vi "ApplicationControlView.vi"(10 "Communicator":refnum<class "Communicator.lvclass">, 11 "UserEvents":refnum<class "UserEvents.lvclass">) -> ()   [LabVIEW 2016, in "M1M3SupportViews.lvlib"]
uses:
  M1M3SupportViews.lvlib
  UserEvents/UserEvents.lvclass
  Communicator/Communicator/Communicator.lvclass
  UserEvents/UserEvents.lvclass/UserEvents.ctl
  DataTypes/Topics/Parts/SummaryStates.ctl
  DataTypes/Topics/CommandStart.ctl
  DataTypes/Topics/Parts/CommandId.ctl
  DataTypes/Topics/CommandEnable.ctl
  DataTypes/Topics/CommandDisable.ctl
  DataTypes/Topics/CommandStandby.ctl
  DataTypes/General/ShutdownEvent.ctl
  DataTypes/Topics/CommandExit.ctl
  DataTypes/Topics/M1M3SupportTopics.lvlib
  DataTypes/General/M1M3SupportGeneral.lvlib
panel:
  in  "Exit":bool
  in  "Shutdown":bool
  in  "Standby":bool
  in  "Disable":bool
  in  "Enable":bool
  in  "Start":bool
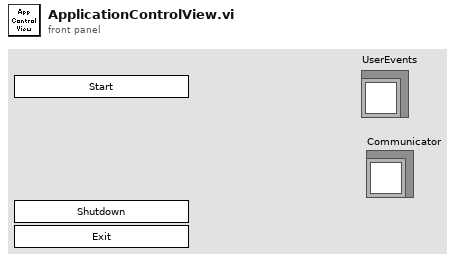
[diagram p1: front panel]
types:
  T1 = typedef "M1M3SupportTopics.lvlib/SummaryStates.ctl" = enum16{"OfflineState", "StandbyState", "DisabledState", "EnabledState", "FaultState"}
  T2 = typedef "M1M3SupportTopics.lvlib/CommandStart.ctl" = cluster{"CommandId":T3, "Start":bool, "SettingToApply":string}
  T3 = typedef "M1M3SupportTopics.lvlib/CommandId.ctl" = i32
  T4 = typedef "M1M3SupportTopics.lvlib/CommandEnable.ctl" = cluster{"CommandId":T3, "Enable":bool}
  T5 = typedef "M1M3SupportTopics.lvlib/CommandDisable.ctl" = cluster{"CommandId":T3, "Disable":bool}
  T6 = typedef "M1M3SupportTopics.lvlib/CommandStandby.ctl" = cluster{"CommandId":T3, "Standby":bool}
  T7 = typedef "M1M3SupportGeneral.lvlib/ShutdownEvent.ctl" = cluster{"Shutdown":bool}
  T8 = typedef "M1M3SupportTopics.lvlib/CommandExit.ctl" = cluster{"CommandId":T3, "Exit":bool}
  T9 = typedef "M1M3SupportTypes.lvlib/SummaryStates.ctl" = enum16{"OfflineState", "StandbyState", "DisabledState", "EnabledState", "FaultState"}
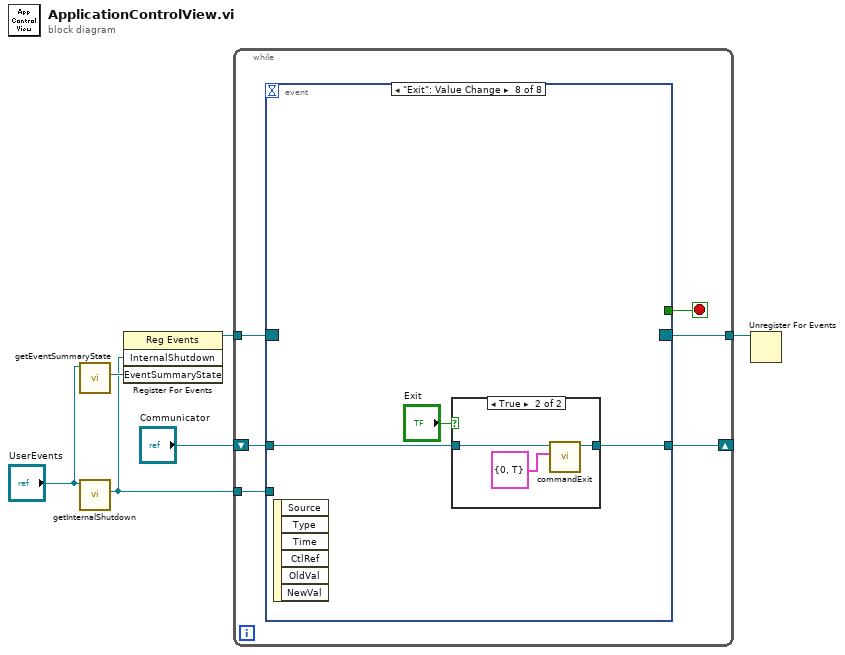
[diagram p0: block diagram]
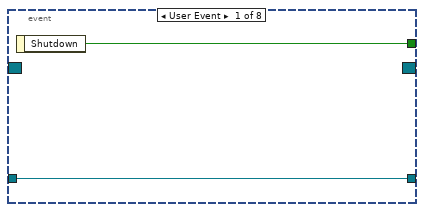
[diagram p2: hidden frame]
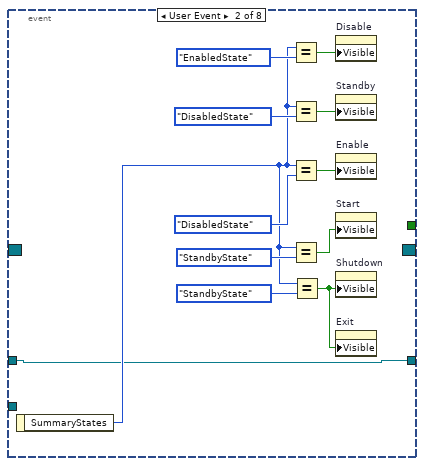
[diagram p3: hidden frame]
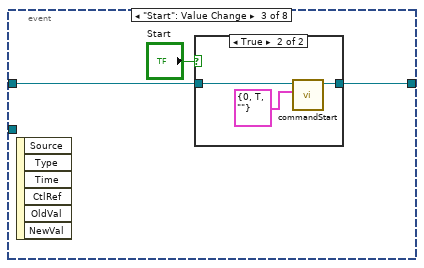
[diagram p4: hidden frame]
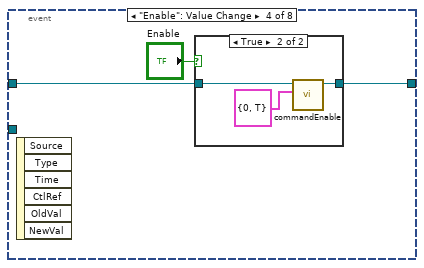
[diagram p6: hidden frame]
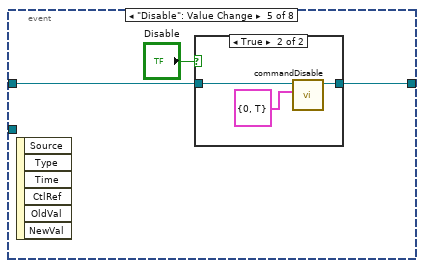
[diagram p8: hidden frame]
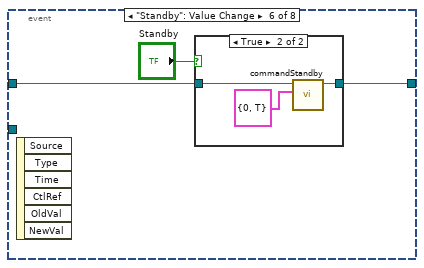
[diagram p10: hidden frame]
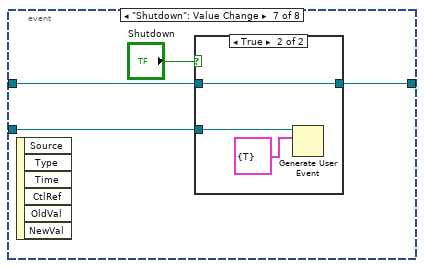
[diagram p12: hidden frame]
diagram:
  n1 = call "getEventSummaryState.vi"("UserEvents in"="UserEvents") -> ("EventSummaryState"=w6:refnum<user-event>)  [unwired: 9 in, 1 out]
  n2 = call "getInternalShutdown.vi"("UserEvents in"="UserEvents") -> ("InternalShutdown"=w1:refnum<user-event>)  [unwired: 9 in, 1 out]
  n3 = register-events(w1, w6) -> (reference out=w5:refnum<event-registration>)  [unwired: 2 in, 1 out]
  n4 = while {
    tunnel: w5 -> [w12]
    tunnel: [w11] -> w4
    shift-right: [w8] -> _
    shift-left: "Communicator" -> [w9]
    tunnel: w1 -> [w7]
    stop <- w10 stop-if-true
    n5 = event shown="[7] \"Exit\": Value Change" {
      selector: w12 -> [_ _ _ _ _ _ _ _]
      dyn-events: [_ _ _ _ _ _ _ _] -> w11
      timeout: _ -> [_ _ _ _ _ _ _ _]
      tunnel: [w14 _ _ _ _ _ _ _] -> w10
      tunnel: w9 -> [w13 w16 w29 w36 w43 w50 w58 w65]
      tunnel: [w13 w16 w28 w35 w42 w49 w57 w64] -> w8
      tunnel: w7 -> [_ _ _ _ _ _ w55 _]
      event User Event {
        n6 = event-data() -> ("Shutdown"=w14:bool)  [unwired: 1 in]
      }
      event User Event {
        n7 = event-data() -> ("SummaryStates"=w17:T9)  [unwired: 1 in]
        n8 = Equal?(x=w17, y=SummaryStates."EnabledState") -> (x = y?=w19:bool)
        n9 = Equal?(x=w17, y=SummaryStates."DisabledState") -> (x = y?=w20:bool)
        n10 = Equal?(x=w17, y=SummaryStates."DisabledState") -> (x = y?=w23:bool)
        n11 = Equal?(x=w17, y=SummaryStates."StandbyState") -> (x = y?=w24:bool)
        n12 = Equal?(x=w17, y=SummaryStates."StandbyState") -> (x = y?=w15:bool)
        n13 = property on="Disable" class="Bool"("Visible"=w19) -> ()  [unwired: 2 in, 2 out]
        n14 = property on="Standby" class="Bool"("Visible"=w20) -> ()  [unwired: 2 in, 2 out]
        n15 = property on="Enable" class="Bool"("Visible"=w23) -> ()  [unwired: 2 in, 2 out]
        n16 = property on="Start" class="Bool"("Visible"=w24) -> ()  [unwired: 2 in, 2 out]
        n17 = property on="Shutdown" class="Bool"("Visible"=w15) -> ()  [unwired: 2 in, 2 out]
        n18 = property on="Exit" class="Bool"("Visible"=w15) -> ()  [unwired: 2 in, 2 out]
      }
      event "Start": Value Change {
        n19 = event-data() -> ()  [unwired: 1 in, 6 out]
        n20 = case shown="True" "Start" {
          tunnel: w29 -> [w30 w32]
          tunnel: [w30 w31] -> w28
          frame False {
          }
          frame True {
            n21 = call-dynamic "commandStart.vi"("CommandStart in"=T2 {"CommandId"=0, "Start"=TRUE, "SettingToApply"=""} ("CommandEnterControl in"), "Communicator in"=w32) -> ("Communicator out"=w31:refnum<class "Communicator.lvclass">)  [unwired: 7 in, 2 out]
          }
        }
      }
      event "Enable": Value Change {
        n22 = event-data() -> ()  [unwired: 1 in, 6 out]
        n23 = case shown="True" "Enable" {
          tunnel: w36 -> [w37 w39]
          tunnel: [w37 w38] -> w35
          frame False {
          }
          frame True {
            n24 = call-dynamic "commandEnable.vi"("CommandEnable in"=T4 {"CommandId"=0, "Enable"=TRUE} ("CommandEnterControl in"), "Communicator in"=w39) -> ("Communicator out"=w38:refnum<class "Communicator.lvclass">)  [unwired: 7 in, 2 out]
          }
        }
      }
      event "Disable": Value Change {
        n25 = event-data() -> ()  [unwired: 1 in, 6 out]
        n26 = case shown="True" "Disable" {
          tunnel: w43 -> [w44 w46]
          tunnel: [w44 w45] -> w42
          frame False {
          }
          frame True {
            n27 = call-dynamic "commandDisable.vi"("CommandDisable in"=T5 {"CommandId"=0, "Disable"=TRUE} ("CommandEnterControl in"), "Communicator in"=w46) -> ("Communicator out"=w45:refnum<class "Communicator.lvclass">)  [unwired: 7 in, 2 out]
          }
        }
      }
      event "Standby": Value Change {
        n28 = event-data() -> ()  [unwired: 1 in, 6 out]
        n29 = case shown="True" "Standby" {
          tunnel: w50 -> [w51 w53]
          tunnel: [w51 w52] -> w49
          frame False {
          }
          frame True {
            n30 = call-dynamic "commandStandby.vi"("CommandStandby in"=T6 {"CommandId"=0, "Standby"=TRUE} ("CommandEnterControl in"), "Communicator in"=w53) -> ("Communicator out"=w52:refnum<class "Communicator.lvclass">)  [unwired: 7 in, 2 out]
          }
        }
      }
      event "Shutdown": Value Change {
        n31 = event-data() -> ()  [unwired: 1 in, 6 out]
        n32 = case shown="True" "Shutdown" {
          tunnel: w58 -> [w59 w60]
          tunnel: [w59 w60] -> w57
          tunnel: w55 -> [_ w62]
          frame False {
          }
          frame True {
            n33 = Generate User Event(user event=w62, event data cluster=T7 {"Shutdown"=TRUE} ("event data")) -> ()  [unwired: 2 in, 2 out]
          }
        }
      }
      event "Exit": Value Change {
        n34 = event-data() -> ()  [unwired: 1 in, 6 out]
        n35 = case shown="True" "Exit" {
          tunnel: w65 -> [w66 w69]
          tunnel: [w66 w68] -> w64
          frame False {
          }
          frame True {
            n36 = call-dynamic "commandExit.vi"("CommandExit in"=T8 {"CommandId"=0, "Exit"=TRUE}, "Communicator in"=w69) -> ("Communicator out"=w68:refnum<class "Communicator.lvclass">)  [unwired: 7 in, 2 out]
          }
        }
      }
    }
  }
  n37 = Unregister For Events(event registration refnum=w4) -> ()  [unwired: 1 in, 1 out]
